vi "in Ursprung setzen.vi"(11 "VI Referenz":refnum<vi>) -> (3 "Referenz (Ausgang)":refnum<vi>)   [LabVIEW 2020, in "allgemeine Sub-VIs.lvlib"]
doc: "Dieses SubVI rückt das Frontpanel in den Ursprung (0,0) zurück.\nEinfach beim initialisieren des Vi´s verwenden.\nVi-ServerReferenz verwenden!"
uses:
  allgemeine Sub-VIs.lvlib
  <vilib>/Utility/miscctls.llb/LVPointTypeDef.ctl
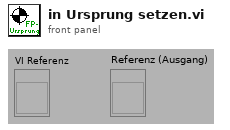
[diagram p1: front panel]
types:
  T1 = typedef "LVPointTypeDef.ctl" = cluster{"Horizontal":i16, "Vertical":i16}
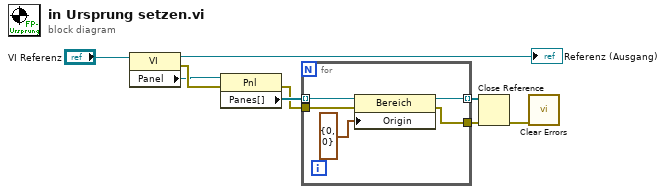
[diagram p0: block diagram]
diagram:
  n1 = property class="VI"(reference="VI Referenz") -> (reference out=→"Referenz (Ausgang)":refnum<vi>, error out=w9:errorcluster, "Panel"=w2:refnum<vi>)  [unwired: 1 in]
  n2 = property class="Pnl"(reference=w2, error in=w9) -> (error out=w7:errorcluster, "Panes[]"=w8:refnum<vi>[])  [unwired: 1 out]
  n3 = for {
    tunnel: w8 -> [w10] mode=indexing
    tunnel: w7 -> [w13]
    tunnel: [w12] -> w6
    tunnel: [w11] -> w5 mode=indexing
    n4 = property class="Bereich"(reference=w10, error in=w13, "Origin"=T1 {"Horizontal"=0, "Vertical"=0} ("Ursprung")) -> (reference out=w11:refnum<vi>, error out=w12:errorcluster)
  }
  n5 = Close Reference(reference=w5, error in (no error)=w6) -> (error out=w3:errorcluster)
  n6 = call <vilib>:"Clear Errors.vi"("error in (no error)"=w3) -> ()  [unwired: 5 in, 2 out]
